vi "event_occurrances.vi"() -> ()   [LabVIEW 2019]
panel:
  out "Numeric":i32
  out "iter":i32
  in  "OK Button":bool
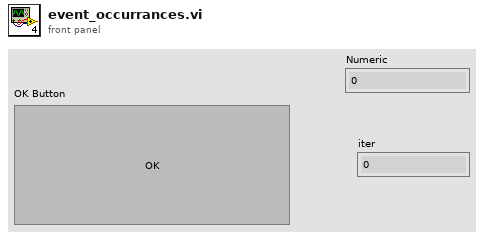
[diagram p1: front panel]
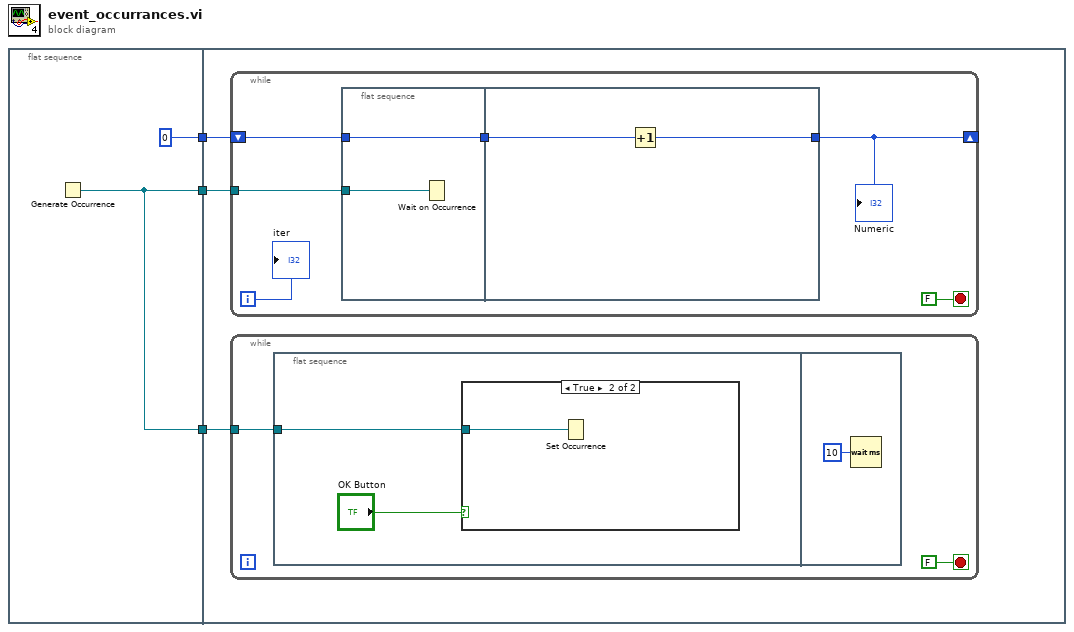
[diagram p0: block diagram]
diagram:
  n1 = flat-sequence {
    tunnel: [w5] -> w3
    tunnel: [w5] -> w2
    tunnel: [0] -> w1
    tunnel: w3 -> [w8]
    tunnel: w2 -> [w7]
    tunnel: w1 -> [w6]
    frame #0 {
      n2 = Generate Occurrence() -> (w5:refnum<k4>)
    }
    frame #1 {
      n3 = while {
        tunnel: w8 -> [w20]
        shift-right: [w15] -> _
        shift-left: w6 -> [w16]
        i -> [w18]
        stop <- FALSE stop-if-true
        n4 = flat-sequence {
          tunnel: w20 -> [w22]
          tunnel: [w21] -> w17
          tunnel: w16 -> [w21]
          tunnel: w17 -> [w24]
          tunnel: [w23] -> w15
          frame #0 {
            n5 = Wait on Occurrence(2:w22) -> ()  [unwired: 2 in, 1 out]
          }
          frame #1 {
            n6 = Increment(x=w24) -> (x+1=w23:i32)
          }
        }
        "iter" <- w18
        "Numeric" <- w15
      }
      n7 = while {
        tunnel: w7 -> [w9]
        stop <- FALSE stop-if-true
        n8 = flat-sequence {
          tunnel: w9 -> [w11]
          frame #0 {
            n9 = case shown="True" "OK Button" {
              tunnel: w11 -> [_ w13]
              frame False {
              }
              frame True {
                n10 = Set Occurrence(w13) -> ()
              }
            }
          }
          frame #1 {
            n11 = Wait (ms)(milliseconds to wait=u32 10) -> ()  [unwired: 1 out]
          }
        }
      }
    }
  }
